vi "CAN_DEBUG_Send.vi"() -> ()   [LabVIEW 2011]
uses:
  _USB_CAN_GLOBAL_.vi
  <vilib>/Utility/file.llb/Read From Spreadsheet File (string).vi
panel:
  in  "channel":u16(ring) items=["通道0", "通道1"]
  in  "TFun":u32
  in  "remote":bool
  in  "ExtFrame":bool
  in  "event":refnum<user-event>
  in  "sendfile":bool
  in  "ID":u32
  in  "Enable":bool
  in  "stop":bool
  in  "Data Inc":bool
  in  "ID Inc":bool
  in  "Cycle":i32=10
  in  "FrameCnt":i32
  in  "data":u8[](array[numeric]) format="%02x"
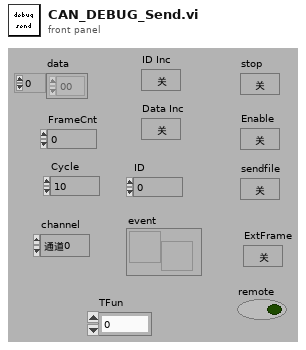
[diagram p1: front panel]
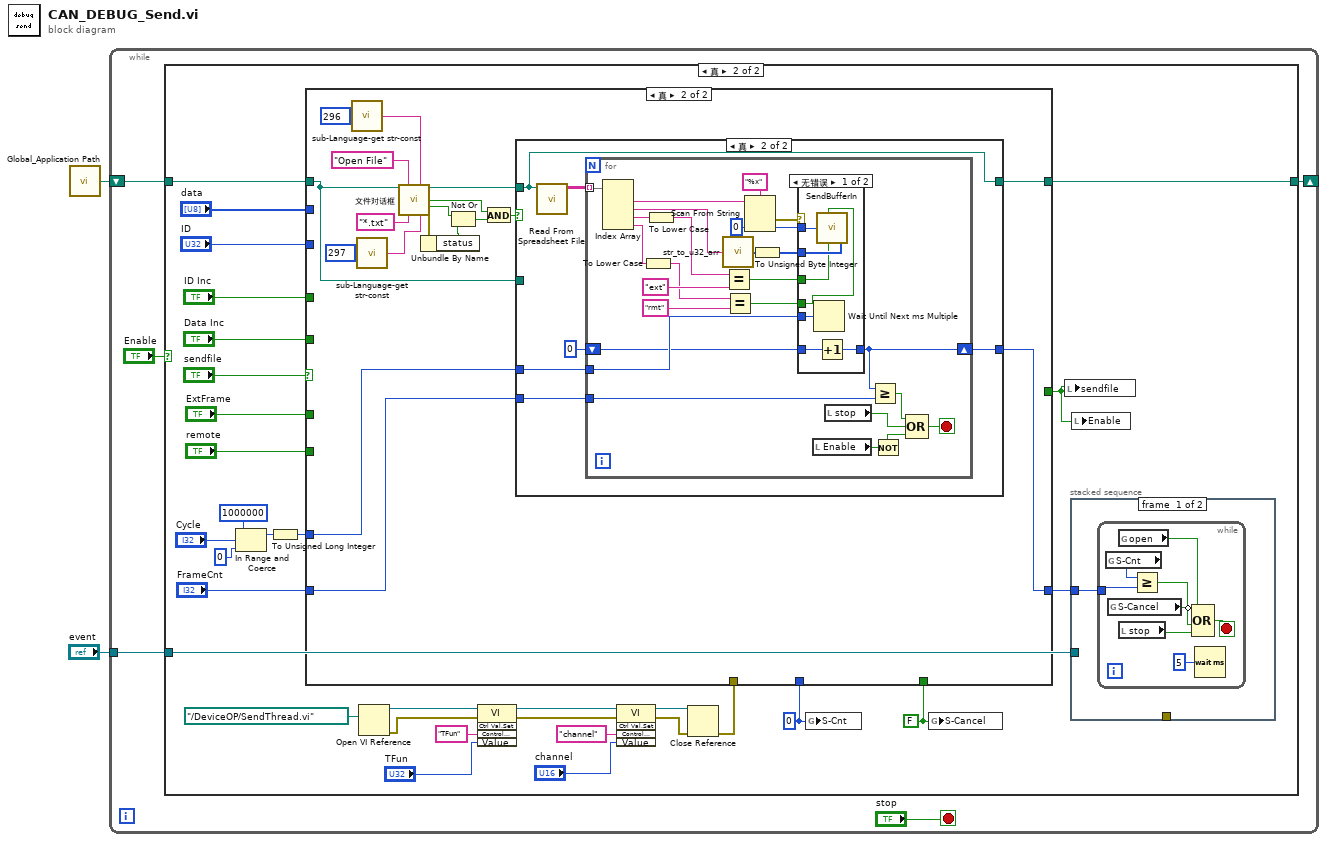
[diagram p0: block diagram]
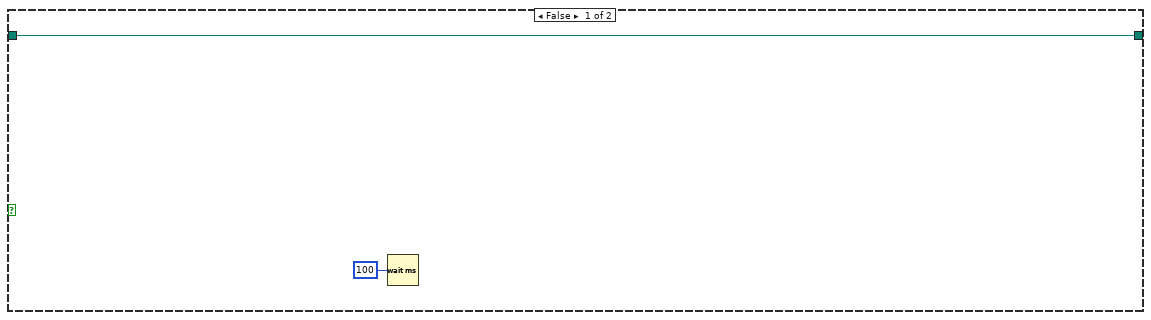
[diagram p2: hidden frame]
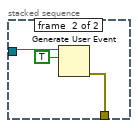
[diagram p3: hidden frame]
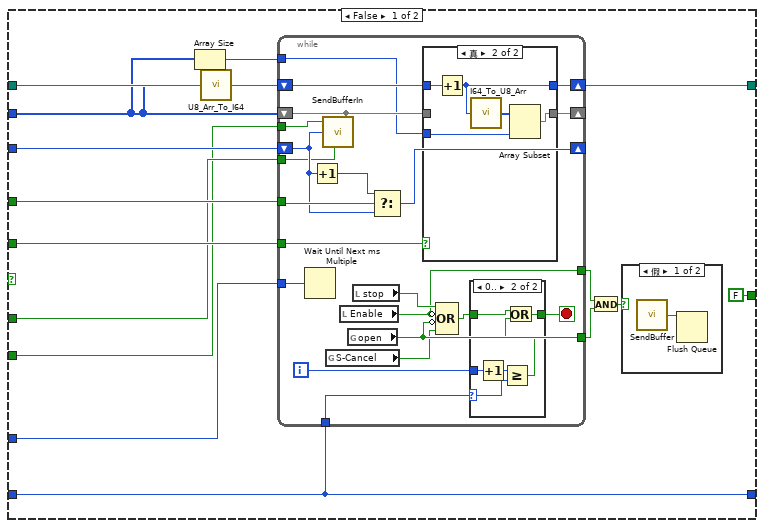
[diagram p4: hidden frame]
diagram:
  n1 = call "Global_Application Path.vi"() -> ("程序路径"=w1:path)  [unwired: 1 in]
  n2 = while {
    tunnel: "event" -> [w5]
    shift-right: [w3] -> _
    shift-left: w1 -> [w4]
    stop <- "stop" stop-if-true
    n3 = case shown="真" "Enable" {
      tunnel: w5 -> [_ w20]
      tunnel: w4 -> [w8 w11]
      tunnel: [w8 w10] -> w3
      frame False {
        n4 = Wait (ms)(milliseconds to wait=u32 100 ("等待时间（毫秒）")) -> ()  [unwired: 1 out]
      }
      frame True {
        w19 = FALSE ("S-Cancel")
        w23 = u32 0 ("S-Cnt")
        n5 = In Range and Coerce(upper limit=1000000 ("上限"), x="Cycle", lower limit=0 ("下限")) -> (coerced(x)=w36:i32)  [unwired: 1 out]
        n6 = To Unsigned Long Integer(number=w36) -> (unsigned 32bit integer=w35:u32)
        n7 = Open VI Reference(vi path=path "../DeviceOP/SendThread.vi" ("VI路径")) -> (vi reference=w28:refnum<vi>, error out=w27:errorcluster)  [unwired: 5 in]
        n8 = invoke class="VI" method="Ctrl Val.Set"(reference=w28, error in=w27, "Control Name"="TFun" ("控件名"), "Value"="TFun") -> (reference out=w18:refnum<vi>, error out=w17:errorcluster)  [unwired: 1 in, 3 out]
        n9 = invoke class="VI" method="Ctrl Val.Set"(reference=w18, error in=w17, "Control Name"="channel" ("控件名"), "Value"="channel") -> (reference out=w16:refnum<vi>, error out=w15:errorcluster)  [unwired: 1 in, 3 out]
        n10 = Close Reference(reference=w16, error in (no error)=w15) -> (error out=w24:errorcluster)
        n11 = case shown="真" "sendfile" {
          tunnel: "FrameCnt" -> [w60 w113]
          tunnel: w35 -> [w61 w112]
          tunnel: "data" -> [w55 _]
          tunnel: "ID" -> [w67 _]
          tunnel: "ID Inc" -> [w66 _]
          tunnel: "Data Inc" -> [w65 _]
          tunnel: [FALSE ("Enable") _] -> w22
          tunnel: "ExtFrame" -> [w63 _]
          tunnel: "remote" -> [w62 _]
          tunnel: w24 -> [_ _]
          tunnel: w23 -> [_ _]
          tunnel: [w60 w111] -> w21
          tunnel: w19 -> [_ _]
          tunnel: w11 -> [w68 w109]
          tunnel: [w68 w110] -> w10
          frame False {
            n12 = Array Size(array=w55) -> (size(s)=w54:i32)
            n13 = call "U8_Arr_To_I64.vi"("data"=w55) -> ("I64"=w56:i64)
            n14 = while {
              shift-right: [w82] -> _
              shift-left: w55 -> [w83]
              shift-right: [w85] -> _
              shift-left: w67 -> [w86]
              tunnel: w66 -> [w88]
              tunnel: w65 -> [w84]
              tunnel: w61 -> [w89]
              shift-right: [w80] -> _
              shift-left: w56 -> [w81]
              tunnel: w63 -> [w78]
              tunnel: w62 -> [w77]
              tunnel: [w76] -> w58
              tunnel: w60 -> [w75]
              tunnel: [w71] -> w59
              tunnel: w54 -> [w69]
              i -> [w72]
              stop <- w73 stop-if-true
              n15 = Wait Until Next ms Multiple(millisecond multiple=w89) -> ()  [unwired: 1 out]
              n16 = Increment(x=w86) -> (x+1=w87:u32)
              n17 = call "SendBufferIn.vi"("remote"=w77, "ID"=w86, "ExtFrame"=w78, "数据"=w83) -> ()  [unwired: 2 in]
              n18 = global read "_USB_CAN_GLOBAL_.vi" "S-Cancel"() -> (w70:bool)
              n19 = local read "Enable"() -> (w71:bool)
              n20 = global read "_USB_CAN_GLOBAL_.vi" "open"() -> (w76:bool)
              n21 = local read "stop"() -> (w79:bool)
              n22 = Select(t=w87, s=w88, f=w86) -> (s? t:f=w85:u32)
              n23 = case shown="真" w84 {
                tunnel: w83 -> [w98 _]
                tunnel: [w98 w99] -> w82
                tunnel: w81 -> [w97 w103]
                tunnel: [w97 w102] -> w80
                tunnel: w69 -> [_ w100]
                frame False {
                }
                frame True {
                  n24 = Increment(x=w103) -> (x+1=w102:i64)
                  n25 = call "I64_To_U8_Arr.vi"("U64"=w102) -> ("data"=w101:u8[])
                  n26 = Array Subset(array=w101, length=w100) -> (w99:u8[])  [unwired: 1 in]
                }
              }
              n27 = Compound Arithmetic op=OR(w79, invert w71, invert w76, w70) -> (w74:bool)
              n28 = case shown="0.." w75 {
                selector: w75 -> [_ w94]
                tunnel: w74 -> [w90 w92]
                tunnel: [w90 w93] -> w73
                tunnel: w72 -> [_ w96]
                frame -1, Default {
                }
                frame 0.. {
                  n29 = Increment(x=w96) -> (x+1=w95:i32)
                  n30 = Greater Or Equal?(x=w95, y=w94) -> (x >= y?=w91:bool)
                  n31 = Or(x=w92, y=w91) -> (x .or. y?=w93:bool)
                }
              }
            }
            n32 = And(x=w59, y=w58) -> (x .and. y?=w57:bool)
            n33 = case shown="假" w57 {
              frame False {
                n34 = call "SendBuffer.vi"() -> ("VCI_CAN_BUF_T"=w104:refnum<queue>)  [unwired: 1 in]
                n35 = Flush Queue(queue=w104) -> ()  [unwired: 1 in, 3 out]
              }
              frame True {
              }
            }
          }
          frame True {
            n36 = call "sub-Language-get str-const.vi"("sid"=u32 296) -> ("str"=w107:string)
            n37 = call "sub-Language-get str-const.vi"("sid"=u32 297) -> ("str"=w105:string)
            n38 = call "文件对话框"("start path"=w109, "prompt"="Open File", "button label"=w107, "pattern (all files)"="*.txt", "pattern label"=w105) -> ("selected path"=w114:path, "exists"=w116:bool, "cancelled"=w118:bool, "error out"=w120:errorcluster)  [unwired: 7 in]
            n39 = Unbundle By Name(w120) -> ("status"=w119:bool)
            n40 = Not Or(1:w119, 2:w118) -> (0:w117:bool)
            n41 = And(x=w116, y=w117) -> (x .and. y?=w115:bool)
            n42 = case shown="真" w115 {
              tunnel: w114 -> [_ w124]
              tunnel: w113 -> [_ w127]
              tunnel: w112 -> [_ w129]
              tunnel: [_ w125] -> w111
              tunnel: [w123 w124] -> w110
              tunnel: w109 -> [w123 _]
              frame False {
              }
              frame True {
                n43 = call-poly <vilib>:"Read From Spreadsheet File.vi"("file path (dialog if empty)"=w124) -> ("all rows"=w128:string[][])  [unwired: 6 in, 4 out]
                n44 = for {
                  tunnel: w128 -> [w155] mode=indexing
                  tunnel: w129 -> [w146]
                  tunnel: w127 -> [w131]
                  shift-right: [w132] -> w125
                  shift-left: 0 -> [w133]
                  stop <- w143 stop-if-true
                  n45 = Index Array(array=w155) -> (element #1=w154:string, element #2=w151:string, element #3=w141:string, element #4=w138:string)  [unwired: 4 in]
                  n46 = To Lower Case(string=w138) -> (all lower case string=w135:string)
                  n47 = To Lower Case(string=w141) -> (all lower case string=w136:string)
                  n48 = call "str_to_u32_arr.vi"("string"=w151) -> ("array"=w150:u32[])
                  n49 = Equal?(x=w136, y="ext") -> (x = y?=w140:bool)
                  n50 = Equal?(x=w135, y="rmt") -> (x = y?=w134:bool)
                  n51 = Scan From String(format string="%x" ("格式字符串"), input string=w154, default 1=u32 0) -> (error out=w149:errorcluster, output 1=w148:u32)  [unwired: 2 in, 2 out]
                  n52 = To Unsigned Byte Integer(number=w150) -> (unsigned 8bit integer=w147:u8[])
                  n53 = case shown="无错误" w149 {
                    tunnel: w148 -> [w162 _]
                    tunnel: w147 -> [w161 _]
                    tunnel: w146 -> [w160 _]
                    tunnel: w140 -> [w159 _]
                    tunnel: w134 -> [w158 _]
                    tunnel: w133 -> [w157 w163]
                    tunnel: [w156 w163] -> w132
                    frame No Error {
                      n54 = Wait Until Next ms Multiple(millisecond multiple=w160) -> ()  [unwired: 1 out]
                      n55 = call "SendBufferIn.vi"("remote"=w158, "ID"=w162, "ExtFrame"=w159, "数据"=w161) -> ()  [unwired: 2 in]
                      n56 = Increment(x=w157) -> (x+1=w156:i32)
                    }
                    frame Error {
                    }
                  }
                  n57 = local read "Enable"() -> (w144:bool)
                  n58 = local read "stop"() -> (w145:bool)
                  n59 = Greater Or Equal?(x=w132, y=w131) -> (x >= y?=w130:bool)
                  n60 = Not(x=w144) -> (.not. x?=w142:bool)
                  n61 = Compound Arithmetic op=OR(w130, w145, w142) -> (w143:bool)
                }
              }
            }
          }
        }
        n62 = global write "_USB_CAN_GLOBAL_.vi" "S-Cnt"(w23) -> ()
        n63 = global write "_USB_CAN_GLOBAL_.vi" "S-Cancel"(w19) -> ()
        n64 = local write "sendfile"(w22) -> ()
        n65 = stacked-sequence {
          tunnel: w21 -> [w42 _]
          tunnel: w20 -> [_ w53]
          tunnel: [_ w51] -> _
          frame #0 {
            n66 = while {
              tunnel: w42 -> [w49]
              stop <- w45 stop-if-true
              n67 = global read "_USB_CAN_GLOBAL_.vi" "S-Cnt"() -> (w48:i64)
              n68 = global read "_USB_CAN_GLOBAL_.vi" "S-Cancel"() -> (w44:bool)
              n69 = global read "_USB_CAN_GLOBAL_.vi" "open"() -> (w43:bool)
              n70 = local read "stop"() -> (w47:bool)
              n71 = Greater Or Equal?(x=w48, y=w49) -> (x >= y?=w46:bool)
              n72 = Compound Arithmetic op=OR(invert w43, w44, w46, w47) -> (w45:bool)
              n73 = Wait (ms)(milliseconds to wait=u32 5 ("等待时间（毫秒）")) -> ()  [unwired: 1 out]
            }
          }
          frame #1 {
            n74 = Generate User Event(user event=w53, event data cluster=TRUE ("事件数据")) -> (error out=w51:errorcluster)  [unwired: 1 in, 1 out]
          }
        }
        n75 = local write "Enable"(w22) -> ()
      }
    }
  }
